vi "index_five_axes.vi"(8 "x_index":i32, 11 "graph_data":cluster{"array type (2D Dbl)":dbl[], dbl[]}[](array[cluster])) -> (0 "Y4":dbl, 1 "Y3":dbl, 2 "Y2":dbl, 3 "Y1":dbl, 4 "Y5":dbl, 5 "X":dbl)   [LabVIEW 2025]
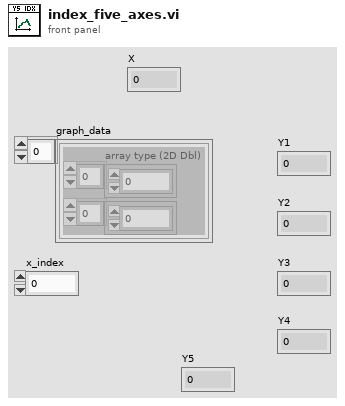
[diagram p1: front panel]
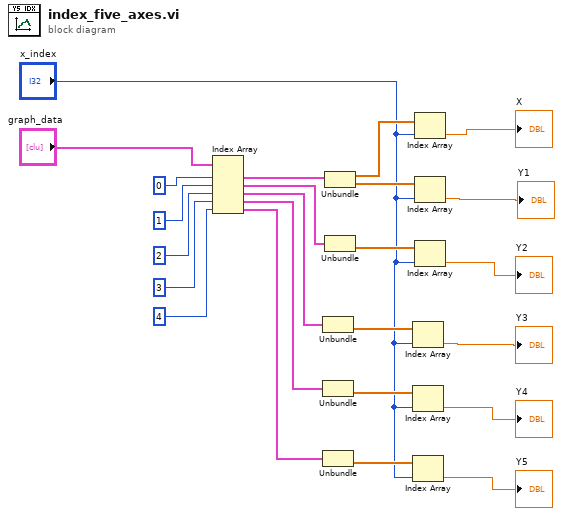
[diagram p0: block diagram]
diagram:
  n1 = Index Array(array="graph_data", index #1=0 ("index"), index #2=1 ("index"), index #3=2 ("index"), index #4=3 ("index"), index #5=4 ("index")) -> (element #1=w18:cluster{"array type (2D Dbl)":dbl[], dbl[]}, element #2=w15:cluster{"array type (2D Dbl)":dbl[], dbl[]}, element #3=w6:cluster{"array type (2D Dbl)":dbl[], dbl[]}, element #4=w5:cluster{"array type (2D Dbl)":dbl[], dbl[]}, element #5=w1:cluster{"array type (2D Dbl)":dbl[], dbl[]})
  n2 = Unbundle(w6) -> (w11:dbl[])  [unwired: 1 out]
  n3 = Unbundle(w5) -> (w10:dbl[])  [unwired: 1 out]
  n4 = Unbundle(w1) -> (w3:dbl[])  [unwired: 1 out]
  n5 = Unbundle(w18) -> ("array type (2D Dbl)"=w20:dbl[], w17:dbl[])
  n6 = Unbundle(w15) -> (w16:dbl[])  [unwired: 1 out]
  n7 = Index Array(array=w11, index="x_index") -> (element=→"Y3":dbl)
  n8 = Index Array(array=w10, index="x_index") -> (element=→"Y4":dbl)
  n9 = Index Array(array=w3, index="x_index") -> (element=→"Y5":dbl)
  n10 = Index Array(array=w20, index="x_index") -> (element=→"X":dbl)
  n11 = Index Array(array=w17, index="x_index") -> (element=→"Y1":dbl)
  n12 = Index Array(array=w16, index="x_index") -> (element=→"Y2":dbl)
